vi "1D Path Array_Sort and Delete Repeating Sells.vi"(2 "1D Path Array.In":path[](array[path])) -> (6 "1D Path Array.Out":path[](array[path]))   [LabVIEW 2020]
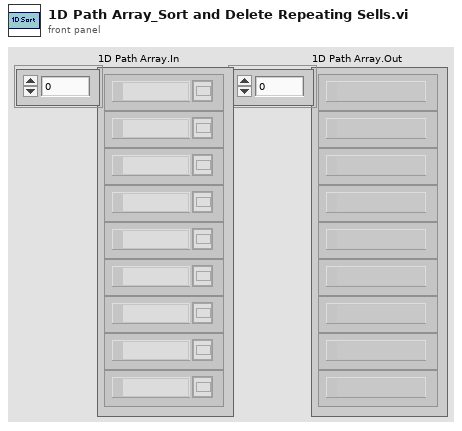
[diagram p1: front panel]
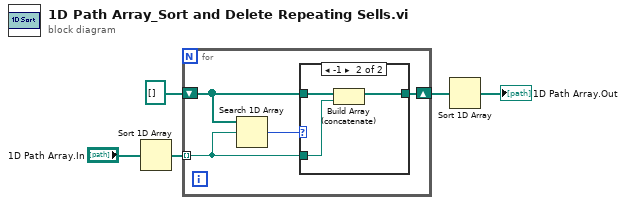
[diagram p0: block diagram]
diagram:
  n1 = Sort 1D Array(array="1D Path Array.In") -> (sorted array=w3:path[])
  n2 = for {
    tunnel: w3 -> [w7] mode=indexing
    shift-right: [w6] -> w5
    shift-left: path[] [] ("sorted array") -> [w8]
    n3 = Search 1D Array(1D array=w8, element=w7) -> (index of element=w9:i32)  [unwired: 1 in]
    n4 = case shown="-1" w9 {
      tunnel: w8 -> [w10 w13]
      tunnel: w7 -> [_ w12]
      tunnel: [w10 w11] -> w6
      frame 0, Default {
      }
      frame -1 {
        n5 = Build Array (concatenate)(w13, w12) -> (w11:path[])
      }
    }
  }
  n6 = Sort 1D Array(array=w5) -> (sorted array=→"1D Path Array.Out":path[])
